vi "XNET UDP Socket Write (Binary).vi"(5 "remote port":u16, 7 "remote address":string, 8 "error in":errorcluster, 9 "timeout ms (25000)":i32=25000, 10 "data":u8[](array[numeric]), 11 "socket in":refnum<k20>) -> (0 "error out":errorcluster, 3 "socket out":refnum<k20>)   [LabVIEW 2018]
doc: "Writes binary data to a UDP network connection."
uses:
  nixlvapi.dll
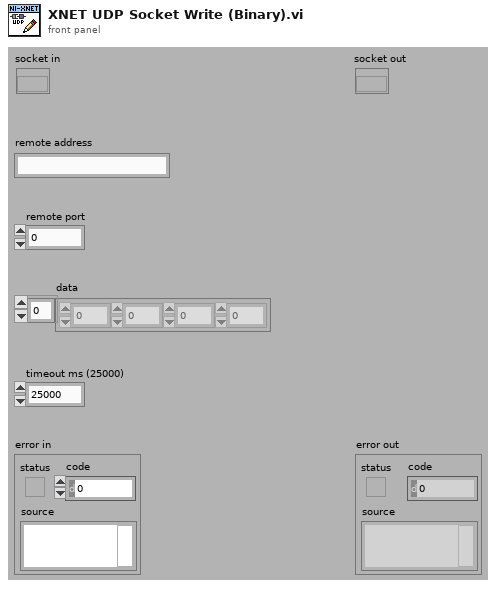
[diagram p1: front panel]
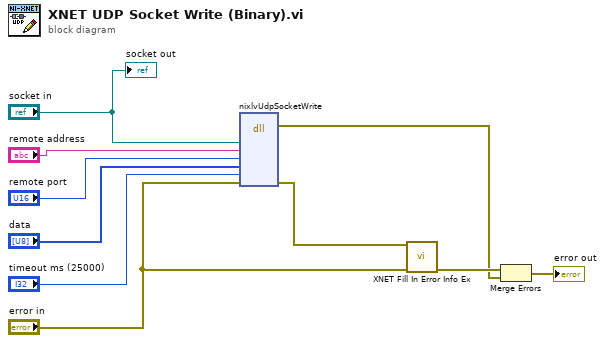
[diagram p0: block diagram]
diagram:
  n1 = dll-call lib="nixlvapi.*" fn="nixlvUdpSocketWrite" label="Call Library"("socketRef"="socket in", "remoteAddress"="remote address", "remotePort"="remote port", "lvData"="data", "timeoutMs"="timeout ms (25000)", "errorInOut"="error in") -> (error out=w8:errorcluster, "errorInOut"=w10:errorcluster)  [unwired: 3 in, 7 out]
  n2 = call "XNET Fill In Error Info Ex.vi"("error xnet"=w10, "error in"="error in") -> ("error out"=w9:errorcluster)  [unwired: 13 in]
  n3 = Merge Errors(w9, w8) -> (→"error out":errorcluster)
  "socket out" <- "socket in"
